vi "Untitled 8.vi"() -> ()   [LabVIEW 2012]
uses:
  <vilib>/addons/database/Connection.llb/DB Tools Open Connec (Path).vi
  <vilib>/addons/database/Connection.llb/Conn Execute.vi
  <vilib>/addons/database/Recordset.llb/Rec Fetch String Data (R).vi
  <vilib>/addons/database/Recordset.llb/Rec Destroy - Connection.vi
  <vilib>/addons/database/Recordset.llb/Rec Fetch Recordset Data (R).vi
  <vilib>/addons/database/_DB Variant To Data/Database Variant To Data.xnode
  <vilib>/addons/database/NI_Database_API.lvlib
panel:
  out "Array":string[][](array[string])
  in  "String 2":string
  in  "String":string="2015-03-23 20:00:00.000"
  out "error out":errorcluster
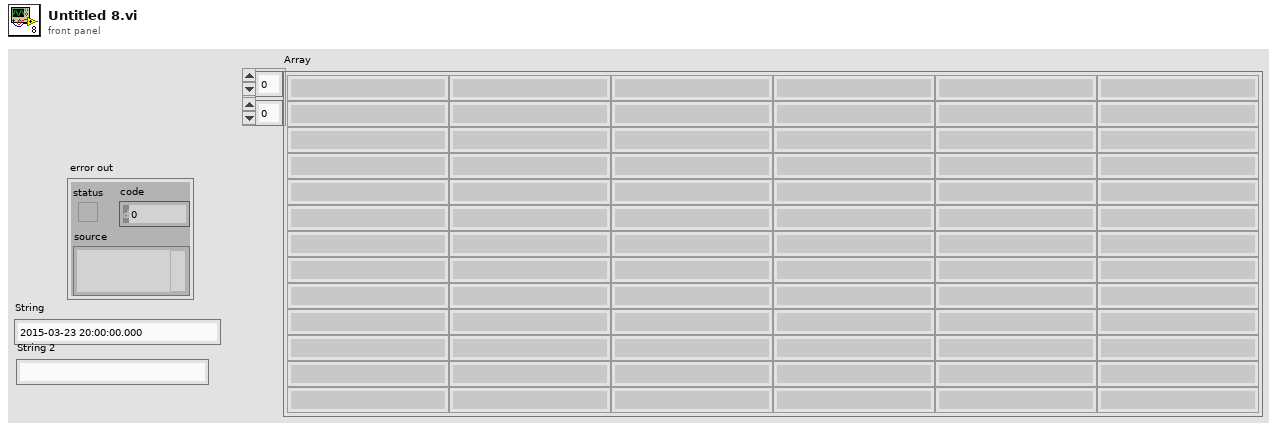
[diagram p1: front panel]
types:
  T1 = typedef "NI_Database_API.lvlib/Conn ObjectReference.ctl" = refnum<k1>
  T2 = typedef "NI_Database_API.lvlib/Rec ObjectReference.ctl" = refnum<k1>
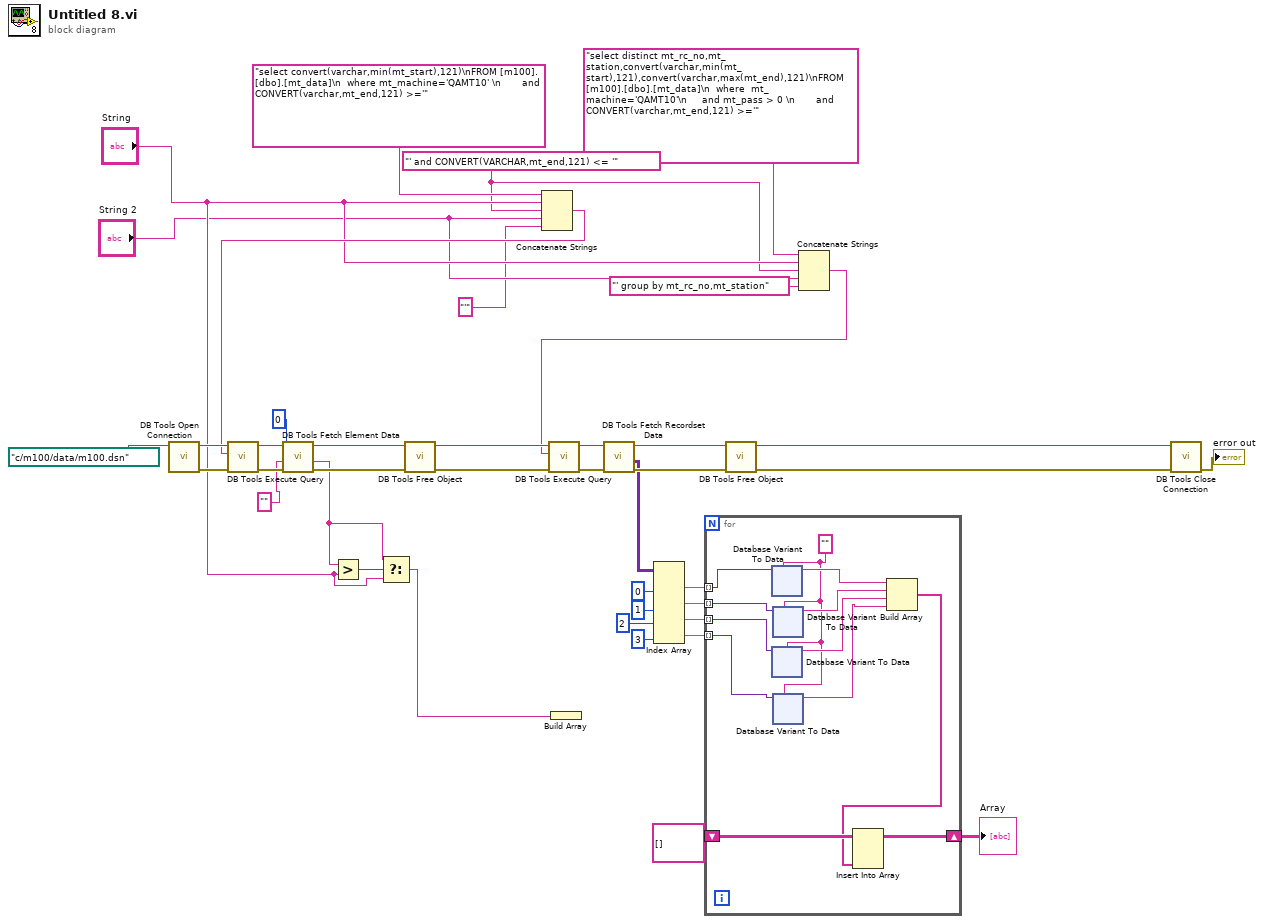
[diagram p0: block diagram]
diagram:
  w11 = "' and CONVERT(VARCHAR,mt_end,121) <= '" ("string")
  n1 = call-poly <vilib>:"DB Tools Open Connection.vi"("connection information"=path "c:/m100/data/m100.dsn") -> ("error out"=w38:errorcluster, "connection reference"=w41:T1)  [unwired: 7 in]
  n2 = Concatenate Strings("select convert(varchar,min(mt_start),121)\nFROM [m100].[dbo].[mt_data]\n  where mt_machine='QAMT10' \n       and CONVERT(varchar,mt_end,121) >='", "String", w11, "String 2", "'" ("string")) -> (w26:string)
  n3 = call-poly <vilib>:"DB Tools Execute Query.vi"("error in (no error)"=w38, "SQL query"=w26, "connection reference"=w41) -> ("error out"=w37:errorcluster, "recordset reference"=w40:T2)  [unwired: 5 in]
  n4 = call-poly <vilib>:"DB Tools Fetch Element Data.vi"("error in (no error)"=w37, "type"="", "column index"=0, "recordset reference"=w40) -> ("error out"=w36:errorcluster, "data"=w22:string, "recordset reference out"=w39:T2)  [unwired: 3 in]
  n5 = Greater?(x=w22, y="String") -> (0:w23:bool)
  n6 = Select(t=w22, s=w23, f="String") -> (s? t:f=w18:string)
  n7 = call-poly <vilib>:"DB Tools Free Object.vi"("error in (no error)"=w36, "recordset reference"=w39) -> ("error out"=w28:errorcluster, "connection reference"=w29:T1)  [unwired: 8 in]
  n8 = Build Array(w18) -> ()  [unwired: 1 out]
  n9 = Concatenate Strings("select distinct mt_rc_no,mt_station,convert(varchar,min(mt_start),121),convert(varchar,max(mt_end),121)\nFROM [m100].[dbo].[mt_data]\n  where  mt_machine='QAMT10'\n     and mt_pass > 0 \n       and CONVERT(varchar,mt_end,121) >='", "String", w11, "String 2", "' group by mt_rc_no,mt_station" ("string")) -> (w16:string)
  n10 = call-poly <vilib>:"DB Tools Execute Query.vi"("error in (no error)"=w28, "SQL query"=w16, "connection reference"=w29) -> ("error out"=w31:errorcluster, "recordset reference"=w33:T2)  [unwired: 5 in]
  n11 = call-poly <vilib>:"DB Tools Fetch Recordset Data.vi"("error in (no error)"=w31, "recordset reference"=w33) -> ("error out"=w30:errorcluster, "recordset data"=w21:variant[][], "recordset reference out"=w32:T2)  [unwired: 3 in]
  n12 = Index Array(array=w21, index (col) #1=0 ("disabled index (col)"), index (col) #2=1 ("index (col)"), index (col) #3=2 ("index (col)"), index (col) #4=3 ("index (col)")) -> (element #1=w19:variant[], element #2=w6:variant[], element #3=w5:variant[], element #4=w2:variant[])  [unwired: 4 in]
  n13 = for {
    tunnel: w19 -> [w53] mode=indexing
    shift-right: [w52] -> w4
    shift-left: string[][] [] -> [w51]
    tunnel: w6 -> [w50] mode=indexing
    tunnel: w5 -> [w49] mode=indexing
    tunnel: w2 -> [w44] mode=indexing
    w42 = ""
    n14 = xnode "Database Variant To Data"("database variant"=w53, "type"=w42) -> ("data"=w48:string)  [unwired: 1 in, 1 out]
    n15 = xnode "Database Variant To Data"("database variant"=w49, "type"=w42) -> ("data"=w46:string)  [unwired: 1 in, 1 out]
    n16 = xnode "Database Variant To Data"("database variant"=w50, "type"=w42) -> ("data"=w47:string)  [unwired: 1 in, 1 out]
    n17 = xnode "Database Variant To Data"("database variant"=w44, "type"=w42) -> ("data"=w43:string)  [unwired: 1 in, 1 out]
    n18 = Build Array(w48, w47, w46, w43) -> (w45:string[])
    n19 = Insert Into Array(array=w51, new element=w45) -> (w52:string[][])  [unwired: 2 in]
  }
  "Array" <- w4
  n20 = call-poly <vilib>:"DB Tools Free Object.vi"("error in (no error)"=w30, "recordset reference"=w32) -> ("error out"=w12:errorcluster, "connection reference"=w13:T1)  [unwired: 8 in]
  n21 = call <vilib>:"DB Tools Close Connection.vi"("error in (no error)"=w12, "connection reference"=w13) -> ("error out"=→"error out":errorcluster)  [unwired: 5 in]
